vi "Pc Robo control test.vi"() -> ()   [LabVIEW 2017]
panel:
  in  "phi 2":dbl
  in  "K2":dbl
  in  "Phi2":dbl(slide) scale=0.0..10.0
  in  "Phi1":dbl(slide) scale=0.0..10.0
  in  "stop":bool
  in  "K2":dbl(slide) scale=-5.0..5.0
  in  "K1":dbl(slide) scale=-5.0..5.0
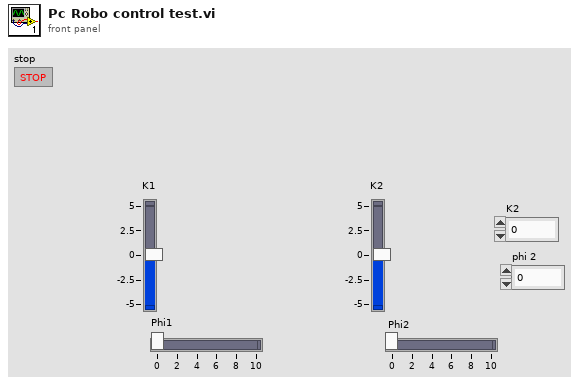
[diagram p1: front panel]
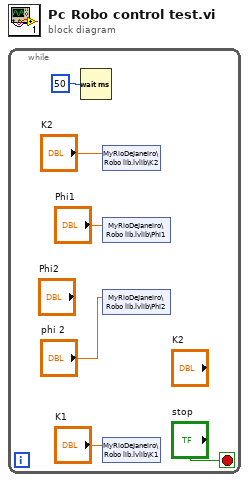
[diagram p0: block diagram]
diagram:
  n1 = while {
    stop <- "stop" stop-if-true
    n2 = Wait (ms)(milliseconds to wait=u32 50) -> ()  [unwired: 1 out]
    n3 = shared-variable "MyRioDeJaneiro\\Robo lib.lvlib\\K2"("K2") -> ()  [unwired: 1 in, 1 out]
    n4 = shared-variable "MyRioDeJaneiro\\Robo lib.lvlib\\Phi1"("Phi1") -> ()  [unwired: 1 in, 1 out]
    n5 = shared-variable "MyRioDeJaneiro\\Robo lib.lvlib\\Phi2"("phi 2") -> ()  [unwired: 1 in, 1 out]
    n6 = shared-variable "MyRioDeJaneiro\\Robo lib.lvlib\\K1"("K1") -> ()  [unwired: 1 in, 1 out]
  }
